vi "emi_Tick Count(ms) with err.vi"(11 "error in (no error)":errorcluster) -> (8 "millisecond timer value":u32, 15 "error out":errorcluster)   [LabVIEW 2011]
doc: "Same as Get Tick Count, but with error in and out. \n\nRuns reentrantly, for posible performance boost.\n\nNo change in behavior due to error"
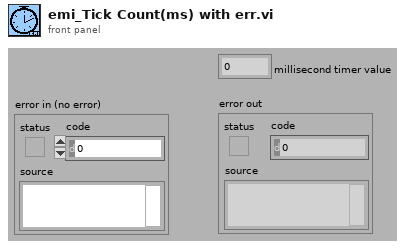
[diagram p1: front panel]
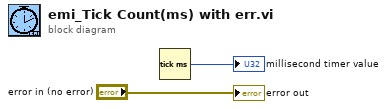
[diagram p0: block diagram]
diagram:
  n1 = Tick Count (ms)() -> (millisecond timer value=→"millisecond timer value":u32)
  "error out" <- "error in (no error)"
